vi "Get Forward Kinematic Matrix.vi"(8 "R4":dbl[](array[numeric]), 9 "R3":dbl[](array[numeric]), 10 "R2":dbl[](array[numeric]), 11 "R1":dbl[](array[numeric])) -> (3 "Real Matrix":T1)   [LabVIEW 2020]
uses:
  <vilib>/Analysis/Matrix/Datatypes/RealMatrix.ctl
  <vilib>/Analysis/Matrix/NI_Matrix.lvlib
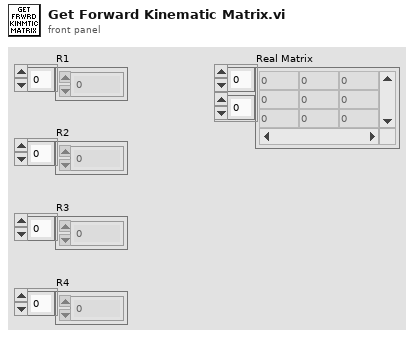
[diagram p1: front panel]
types:
  T1 = typedef "NI_Matrix.lvlib/RealMatrix.ctl" = dbl[][]
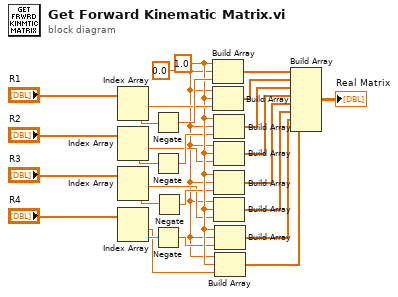
[diagram p0: block diagram]
diagram:
  w1 = 0.0 ("element")
  w15 = 1.0 ("element")
  n1 = Index Array(array="R1") -> (element #1=w17:dbl, element #2=w22:dbl)  [unwired: 2 in]
  n2 = Index Array(array="R2") -> (element #1=w13:dbl, element #2=w12:dbl)  [unwired: 2 in]
  n3 = Index Array(array="R3") -> (element #1=w10:dbl, element #2=w21:dbl)  [unwired: 2 in]
  n4 = Index Array(array="R4") -> (element #1=w8:dbl, element #2=w20:dbl)  [unwired: 2 in]
  n5 = Negate(x=w22) -> (-x=w19:dbl)
  n6 = Negate(x=w12) -> (-x=w14:dbl)
  n7 = Negate(x=w20) -> (-x=w9:dbl)
  n8 = Negate(x=w21) -> (-x=w11:dbl)
  n9 = Build Array(w15, w1, w19) -> (w18:dbl[])
  n10 = Build Array(w1, w15, w17) -> (w16:dbl[])
  n11 = Build Array(w15, w1, w14) -> (w7:dbl[])
  n12 = Build Array(w1, w15, w13) -> (w6:dbl[])
  n13 = Build Array(w15, w1, w11) -> (w5:dbl[])
  n14 = Build Array(w1, w15, w10) -> (w4:dbl[])
  n15 = Build Array(w15, w1, w9) -> (w3:dbl[])
  n16 = Build Array(w1, w15, w8) -> (w2:dbl[])
  n17 = Build Array(w18, w16, w7, w6, w5, w4, w3, w2) -> (→"Real Matrix":T1)
